vi "CFTS-Write State.vi"(0 "State":T1, 11 "error in (no error)":errorcluster) -> (4 "State thru":T1, 15 "error out":errorcluster)   [LabVIEW 2020]
uses:
  CFTS-Experiment State.ctl
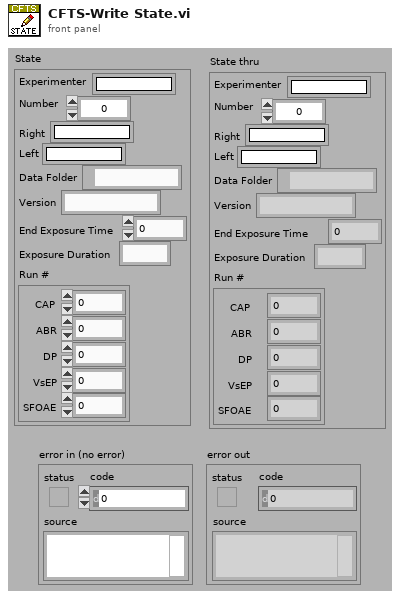
[diagram p1: front panel]
types:
  T1 = typedef "CFTS-Experiment State.ctl" = cluster{"Experimenter":string, "Number":u32, "Right":string, "Left":string, "Data Folder":path, "Version":string, "End Exposure Time":dbl, "Exposure Duration":string, "Run #":cluster{"CAP":i32, "ABR":i32, "DP":i32, "VsEP":i32, "SFOAE":i32}}
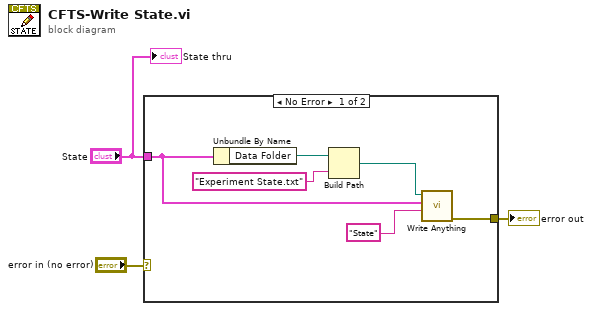
[diagram p0: block diagram]
diagram:
  n1 = case shown="No Error" "error in (no error)" {
    selector: "error in (no error)" -> [_ w10]
    tunnel: "State" -> [w4 _]
    tunnel: [w8 w10] -> w2
    frame No Error {
      n2 = Unbundle By Name(w4) -> ("Data Folder"=w6:path)
      n3 = Build Path(base path=w6, name or relative path="Experiment State.txt" ("subkey")) -> (appended path=w7:path)
      n4 = call "Write Anything.vi"("Section Name (Name of \"Anything\")"="State" ("subkey"), "Anything"=w4, "Path (dialog)"=w7) -> ("Error Out"=w8:errorcluster)  [unwired: 7 in, 1 out]
    }
    frame Error {
    }
  }
  "error out" <- w2
  "State thru" <- "State"
